vi "readFromXMLAzimuth.vi"(8 "error in (no error)":errorcluster, 10 "XML in":string="<Azimuth>\n  <degreesArc>44.33</degreesArc>\n  <minutesArc>33.22</minutesArc>\n  <secondsArc>22.11</secondsArc>\n</Azimuth>") -> (0 "error out":errorcluster)   [LabVIEW 2012]
uses:
  <userlib>/Common/UnitsAndXML/FlattenItemWithUnitToXML/FlattenPlaneAngleToXML/PlaneAngleUnit.ctl
  <userlib>/Common/UnitsAndXML/UnitsAndXML.lvlib
  <userlib>/Common/XML/XMLParser/XMLParser.lvclass
panel:
  in  "degreesArc 2":dbl[unit]=0.7737044574090862
  in  "minutesArc 2":dbl[unit]=0.00966330629187527
  in  "secondsArc 2":dbl[unit]=0.00010719230489331841
  out "Element out":refnum<class "XMLParser.lvclass">
  in  "Element in":refnum<class "XMLParser.lvclass">=refnum
  out "secondsArc":dbl[unit]=0.00010719230489331841
  out "minutesArc":dbl[unit]=0.00966330629187527
  out "degreesArc":dbl[unit]=0.7737044574090862
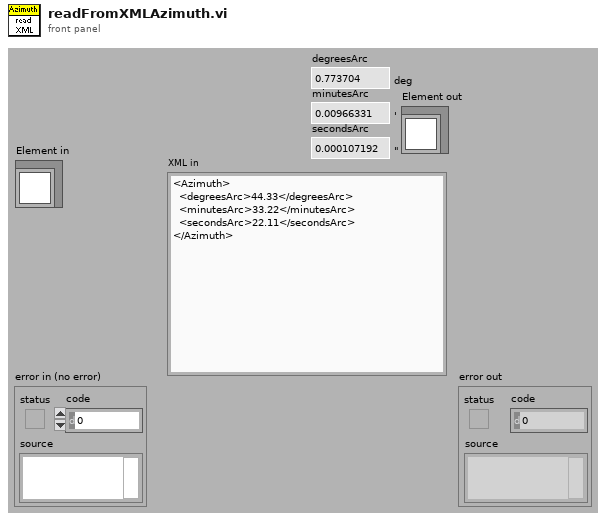
[diagram p1: front panel]
types:
  T1 = typedef "UnitsAndXML.lvlib/PlaneAngleUnit.ctl" = enum16{"rad", "deg", "'", "\""}
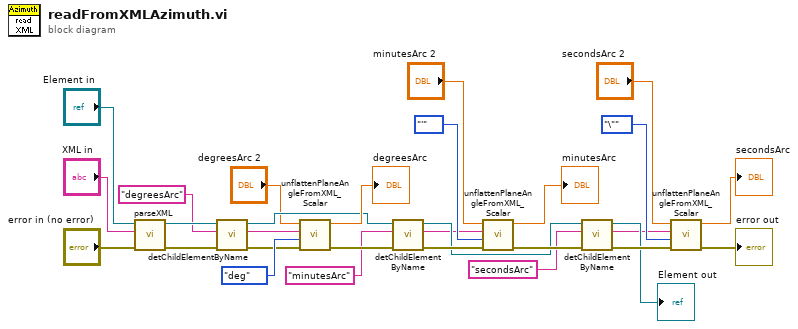
[diagram p0: block diagram]
diagram:
  n1 = call <userlib>:"parseXML.vi"("error in (no error)"="error in (no error)", "XMLString in"="XML in", "Element in"="Element in") -> ("error out"=w19:errorcluster, "Element out"=w20:refnum<class "XMLParser.lvclass">)  [unwired: 7 in]
  n2 = call <userlib>:"detChildElementByName.vi"("error in (no error)"=w19, "childName"="degreesArc" ("ChildName"), "Element in"=w20) -> ("error out"=w14:errorcluster, "childXML"=w5:string, "Element out"=w12:refnum<class "XMLParser.lvclass">)  [unwired: 5 in, 1 out]
  n3 = call <userlib>:"unflattenPlaneAngleFromXML_Scalar.vi"("error in (no error)"=w14, "planeAngleUnitInXML"=PlaneAngleUnit."deg", "xmlString"=w5, "planeAngleForType"="degreesArc 2") -> ("error out"=w15:errorcluster, "planeAngle"=→"degreesArc":dbl[unit])  [unwired: 6 in]
  n4 = call <userlib>:"detChildElementByName.vi"("error in (no error)"=w15, "childName"="minutesArc" ("ChildName"), "Element in"=w12) -> ("error out"=w16:errorcluster, "childXML"=w7:string, "Element out"=w11:refnum<class "XMLParser.lvclass">)  [unwired: 5 in, 1 out]
  n5 = call <userlib>:"unflattenPlaneAngleFromXML_Scalar.vi"("error in (no error)"=w16, "planeAngleUnitInXML"=PlaneAngleUnit."'", "xmlString"=w7, "planeAngleForType"="minutesArc 2") -> ("error out"=w17:errorcluster, "planeAngle"=→"minutesArc":dbl[unit])  [unwired: 6 in]
  n6 = call <userlib>:"detChildElementByName.vi"("error in (no error)"=w17, "childName"="secondsArc" ("ChildName"), "Element in"=w11) -> ("error out"=w13:errorcluster, "childXML"=w9:string, "Element out"=→"Element out":refnum<class "XMLParser.lvclass">)  [unwired: 5 in, 1 out]
  n7 = call <userlib>:"unflattenPlaneAngleFromXML_Scalar.vi"("error in (no error)"=w13, "planeAngleUnitInXML"=PlaneAngleUnit."\"", "xmlString"=w9, "planeAngleForType"="secondsArc 2") -> ("error out"=→"error out":errorcluster, "planeAngle"=→"secondsArc":dbl[unit])  [unwired: 6 in]
